vi "Overall RaF Scripting.vi"() -> ()   [LabVIEW 2017, in "Switch Scripting.lvlib"]
uses:
  Switch Scripting.lvlib
  Routing Channel/Alias Mapping.ctl
  Routing Channel/Connection.ctl
  NationalInstruments.VeriStand.SystemDefinitionAPI
  Routing State.ctl
  github/niveristand-engine-simulation-toolkit-custom-device/Source/Scripting API/Custom Device/Engine Simulation Toolkit Custom Device Settings.ctl
  <vilib>/NI VeriStand/Custom Device API/Custom Device API.lvlib
  <vilib>/NI Veristand/Custom Device API/Set Item Property (String).vi
panel:
  out "All Alias Mappings":T1[](array[typedef])
  out "Alias found":bool
  out "Pin":string
  out "new SDF file":path
  out "error out":errorcluster
  out "error":string
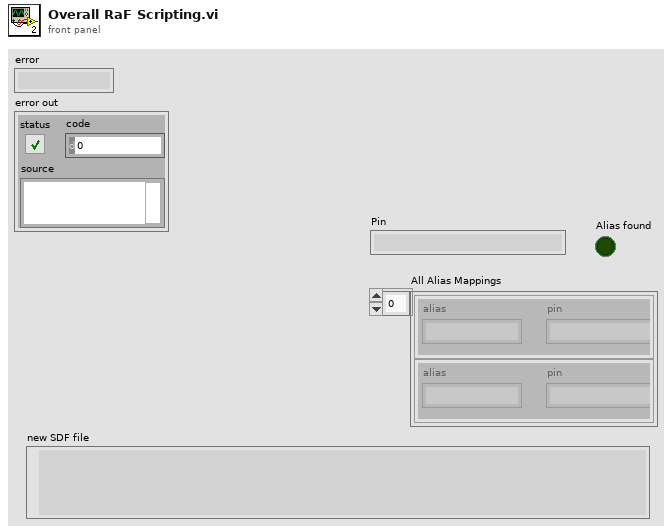
[diagram p1: front panel]
types:
  T1 = typedef "Switch Scripting.lvlib/Alias Mapping.ctl" = cluster{"alias":string, "pin":string}
  T2 = typedef "Switch Scripting.lvlib/Connection.ctl" = cluster{"source":string, "destination":string}
  T3 = typedef "Custom Device API.lvlib/Custom Device Item Ref.ctl" = u64
  T4 = typedef "Switch Scripting.lvlib/Routing State.ctl" = cluster{"name":string, "description":string, "value":i32, "connection list":T2[]}
  T5 = typedef "Engine Simulation Toolkit Scripting API.lvlib/Engine Simulation Toolkit Custom Device Settings.ctl" = cluster{"Name":string, "Execution priority":enum16{"Low", "Medium", "High"}, "Rate decimation":i32, "CPU":i32}
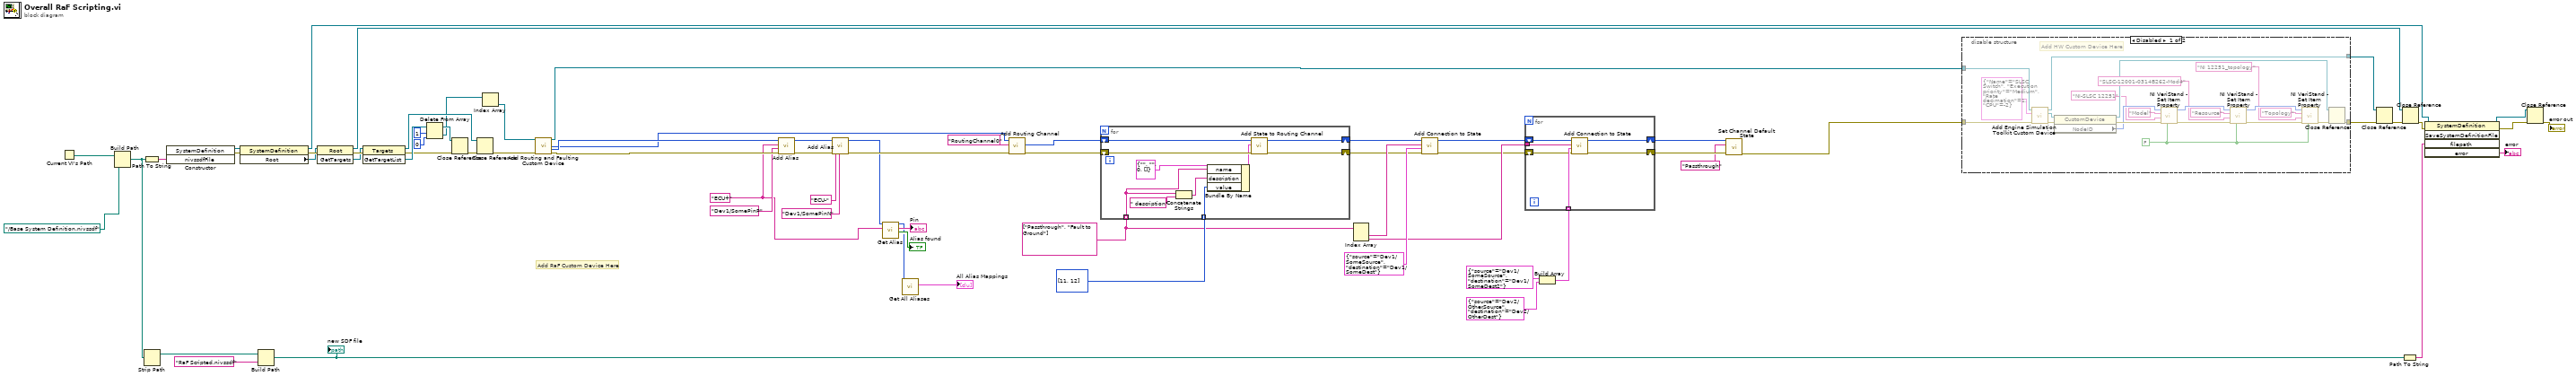
[diagram p0: block diagram]
diagram:
  w25 = "ECU+" ("Property Name")
  w16 = string[] ["Passthrough", "Fault to Ground"] ("names")
  # "Add RaF Custom Device Here"
  n1 = Current VI's Path() -> (path=w42:path)
  n2 = Build Path(base path=w42, name or relative path=path "../Base System Definition.nivssdf" ("Absolute or Relative Path")) -> (appended path=w40:path)
  n3 = Path To String(path=w40) -> (string=w68:string)
  n4 = Strip Path(path=w40) -> (stripped path=w53:path)  [unwired: 1 out]
  n5 = constructor class="SystemDefinition"("nivssdfFile"=w68) -> (reference out=w67:refnum<k24>, error out=w69:errorcluster)  [unwired: 3 in, 2 out]
  n6 = property class="SystemDefinition"(reference=w67, error in=w69) -> (reference out=w54:refnum<k24>, error out=w66:errorcluster, "Root"=w65:refnum<k24>)
  n7 = Build Path(base path=w53, name or relative path="RaF Scripted.nivssdf") -> (appended path=w34:path)
  "new SDF file" <- w34
  n8 = invoke class="Root" method="GetTargets"(reference=w65, error in=w66) -> (reference out=w50:refnum<k24>, error out=w64:errorcluster, "GetTargets"=w63:refnum<k24>)  [unwired: 1 in]
  n9 = invoke class="Targets" method="GetTargetList"(reference=w63, error in=w64) -> (reference out=w56:refnum<k24>, error out=w59:errorcluster, "GetTargetList"=w62:refnum<k24>[])  [unwired: 1 in]
  n10 = Delete From Array(array=w62, length=1, index=0) -> (deleted portion=w55:refnum<k24>[], array with subset deleted=w58:refnum<k24>[])
  n11 = Close Reference(reference=w58, error in (no error)=w59) -> (error out=w57:errorcluster)
  n12 = Close Reference(reference=w56, error in (no error)=w57) -> (error out=w36:errorcluster)
  n13 = Index Array(array=w55) -> (element=w38:refnum<k24>)  [unwired: 1 in]
  n14 = call "Add Routing and Faulting Custom Device.vi"("Target in"=w38, "error in (no error)"=w36) -> ("Target out"=w37:refnum<k24>, "Routes Section Ref"=w20:T3, "Aliases Section Ref"=w33:T3, "error out"=w35:errorcluster)  [unwired: 9 in, 1 out]
  n15 = call "Add Alias.vi"("error in (no error)"=w35, "Pin"="Dev1/SomePinP" ("Property Name"), "Alias"=w25, "Aliases Ref in"=w33) -> ("error out"=w26:errorcluster, "Aliases Ref out"=w27:T3)  [unwired: 6 in]
  n16 = call "Add Alias.vi"("error in (no error)"=w26, "Pin"="Dev1/SomePinN" ("Property Name"), "Alias"="ECU-" ("Property Name"), "Aliases Ref in"=w27) -> ("error out"=w32:errorcluster, "Aliases Ref out"=w22:T3)  [unwired: 6 in]
  n17 = call "Get Alias.vi"("Alias"=w25, "Aliases Ref in"=w22) -> ("Alias found"=→"Alias found":bool, "Pin"=→"Pin":string, "Aliases Ref out"=w21:T3)  [unwired: 6 in, 1 out]
  n18 = call "Get All Aliases.vi"("Aliases Ref in"=w21) -> ("All Alias Mappings"=→"All Alias Mappings":T1[])  [unwired: 7 in, 3 out]
  n19 = call "Add Routing Channel.vi"("error in (no error)"=w32, "Channel Name"="RoutingChannel0" ("Channel"), "Routes Ref in"=w20) -> ("error out"=w17:errorcluster, "Channel Ref"=w19:T3)  [unwired: 6 in, 1 out]
  n20 = for {
    tunnel: w16 -> [w73] mode=indexing
    tunnel: i32[] [11, 12] ("values") -> [w71] mode=indexing
    shift-right: [w77] -> w13
    shift-left: w17 -> [w78]
    shift-right: [w76] -> w12
    shift-left: w19 -> [w79]
    n21 = Concatenate Strings(w73, " description" ("string")) -> (w72:string)
    n22 = Bundle By Name(cluster=T4 {"name"="", "description"="", "value"=0, "connection list"=[]} ("Routing State"), "name"=w73, "description"=w72, "value"=w71) -> (w70:T4)
    n23 = call "Add State to Routing Channel.vi"("error in (no error)"=w78, "Routing State"=w70, "Channel Ref in"=w79) -> ("error out"=w77:errorcluster, "Channel Ref out"=w76:T3)  [unwired: 7 in]
  }
  n24 = Index Array(array=w16) -> (element #1=w15:string, element #2=w9:string)  [unwired: 2 in]
  n25 = call "Add Connection to State.vi"("error in (no error)"=w13, "Connection"=T2 {"source"="Dev1/SomeSource", "destination"="Dev1/SomeDest"}, "State"=w15, "Channel Ref in"=w12) -> ("error out"=w7:errorcluster, "Channel Ref out"=w6:T3)  [unwired: 6 in]
  n26 = Build Array(T2 {"source"="Dev1/SomeSource", "destination"="Dev1/SomeDest2"} ("Connection"), T2 {"source"="Dev2/OtherSource", "destination"="Dev2/OtherDest"} ("Connection")) -> (w8:T2[])
  n27 = for {
    tunnel: w9 -> [w85]
    tunnel: w8 -> [w84] mode=indexing
    shift-right: [w80] -> w5
    shift-left: w6 -> [w82]
    shift-right: [w81] -> w4
    shift-left: w7 -> [w83]
    n28 = call "Add Connection to State.vi"("error in (no error)"=w83, "Connection"=w84, "State"=w85, "Channel Ref in"=w82) -> ("error out"=w81:errorcluster, "Channel Ref out"=w80:T3)  [unwired: 6 in]
  }
  n29 = call "Set Channel Default State.vi"("error in (no error)"=w4, "State"="Passthrough", "Channel Ref in"=w5) -> ("error out"=w1:errorcluster)  [unwired: 7 in, 1 out]
  n30 = disable-structure shown="Disabled" {
    disable-tunnel: w1 -> [w107 _]
    disable-tunnel: w37 -> [w106 w108]
    disable-tunnel: [w95 _] -> w46
    disable-tunnel: [w86 w108] -> w39
    frame Disabled {
      w99 = FALSE ("Binary String (T)")
      # "Add HW Custom Device Here"
      n31 = call "Add Engine Simulation Toolkit Custom Device.vi"("error in (no error)"=w107, "Settings"=T5 {"Name"="SLSC Switch", "Execution priority"=enum."Medium", "Rate decimation"=1, "CPU"=-2}, "Target in"=w106) -> ("error out"=w104:errorcluster, "EST Custom Device"=w103:refnum<k24>, "Target out"=w86:refnum<k24>)  [unwired: 6 in]
      n32 = property class="CustomDevice"(reference=w103, error in=w104) -> (reference out=w94:refnum<k24>, error out=w102:errorcluster, "NodeID"=w101:u64)
      n33 = call-poly <vilib>:"NI VeriStand - Set Item Property.vi"("Binary String (T)"=w99, "error in (no error)"=w102, "Value"="NI-SLSC 12251", "Property Name"="Model", "Item Ref in"=w101) -> ("error out"=w98:errorcluster, "Item Ref out"=w93:T3)  [unwired: 4 in, 1 out]
      n34 = call-poly <vilib>:"NI VeriStand - Set Item Property.vi"("Binary String (T)"=w99, "error in (no error)"=w98, "Value"="SLSC-12001-0314B262-Mod4", "Property Name"="Resource", "Item Ref in"=w93) -> ("error out"=w97:errorcluster, "Item Ref out"=w92:T3)  [unwired: 4 in, 1 out]
      n35 = call-poly <vilib>:"NI VeriStand - Set Item Property.vi"("Binary String (T)"=w99, "error in (no error)"=w97, "Value"="NI 12251_topology", "Property Name"="Topology", "Item Ref in"=w92) -> ("error out"=w96:errorcluster)  [unwired: 4 in, 2 out]
      n36 = Close Reference(reference=w94, error in (no error)=w96) -> (error out=w95:errorcluster)
    }
    frame Enabled {
    }
  }
  n37 = Close Reference(reference=w39, error in (no error)=w46) -> (error out=w45:errorcluster)
  n38 = Path To String(path=w34) -> (string=w51:string)
  n39 = Close Reference(reference=w50, error in (no error)=w45) -> (error out=w44:errorcluster)
  n40 = invoke class="SystemDefinition" method="SaveSystemDefinitionFile"(reference=w54, error in=w44, "filepath"=w51) -> (reference out=w49:refnum<k24>, error out=w43:errorcluster, "error"=→"error":string)  [unwired: 2 in, 2 out]
  n41 = Close Reference(reference=w49, error in (no error)=w43) -> (error out=→"error out":errorcluster)
